vi "GetLayer.vi"(7 "Actor":refnum<class "Actor.lvclass">) -> (3 "Layer":T1)   [LabVIEW 2020, in "jettl.lvlib" / "Base.lvlib" / "Actor.lvclass"]
uses:
  Actor.lvclass
  Actor.lvclass/Actor.ctl
  Msg/Msg.lvclass
  MsgSet.ctl
  jettl.lvlib
  LayerType.ctl
  Layer.ctl
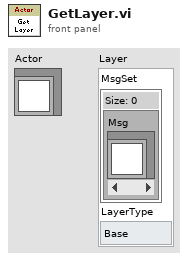
[diagram p1: front panel]
types:
  T1 = typedef "jettl.lvlib/Layer.ctl" = cluster{"MsgSet":T2, "LayerType":T3}
  T2 = typedef "jettl.lvlib/MsgSet.ctl" = set{refnum<class "Msg.lvclass">}
  T3 = typedef "jettl.lvlib/LayerType.ctl" = enum16{"Base", "InnerGlobal", "InnerLocal", "Outer"}
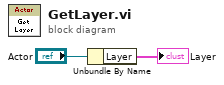
[diagram p0: block diagram]
diagram:
  n1 = Unbundle By Name("Actor") -> ("Layer"=→"Layer":T1)
